vi "Fc_2update_graph.vi"(9 "Cluster in":T1, 10 "Local Mode":enum32{"Resume", "Hold"}(ring), 11 "WaveformGraph in":refnum<vi>) -> (2 "Cluster in 2":T1, 3 "Update Waveform Graph":bool)   [LabVIEW 2021]
doc: "This function updates the waveform graph."
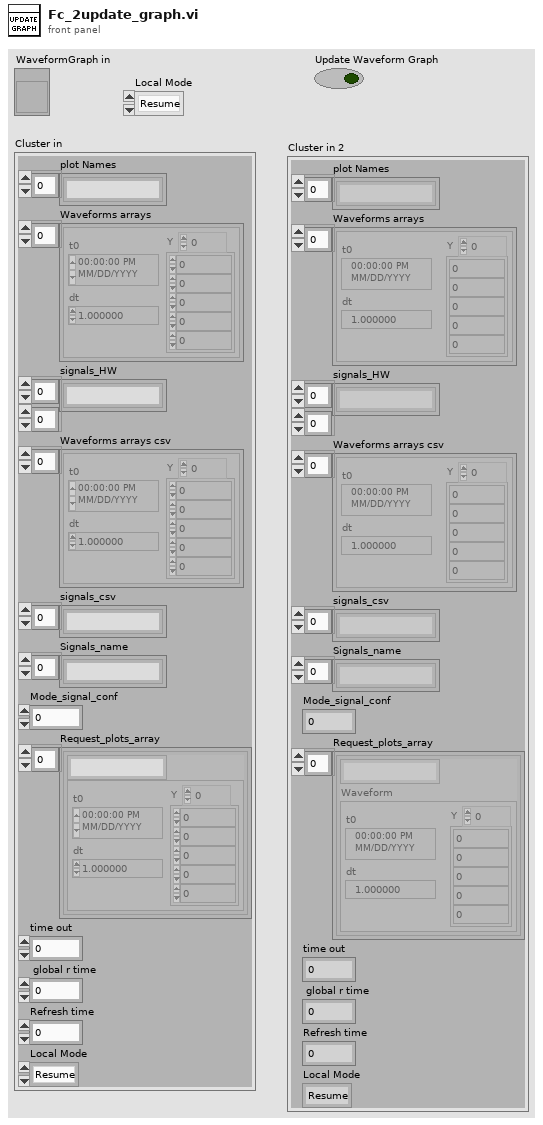
[diagram p1: front panel]
types:
  T1 = cluster{"plot Names":string[], "Waveforms arrays":waveform(dbl)[], "signals_HW":string[][], "Waveforms arrays csv":waveform(dbl)[], "signals_csv":string[], "Signals_name":string[], "Mode_signal_conf":u8, "Request_plots_array":cluster{string, "Waveform":waveform(dbl)}[], "time out":i32, " global r time":u32, "Refresh time":u32, "Local Mode":enum32{"Resume", "Hold"}}
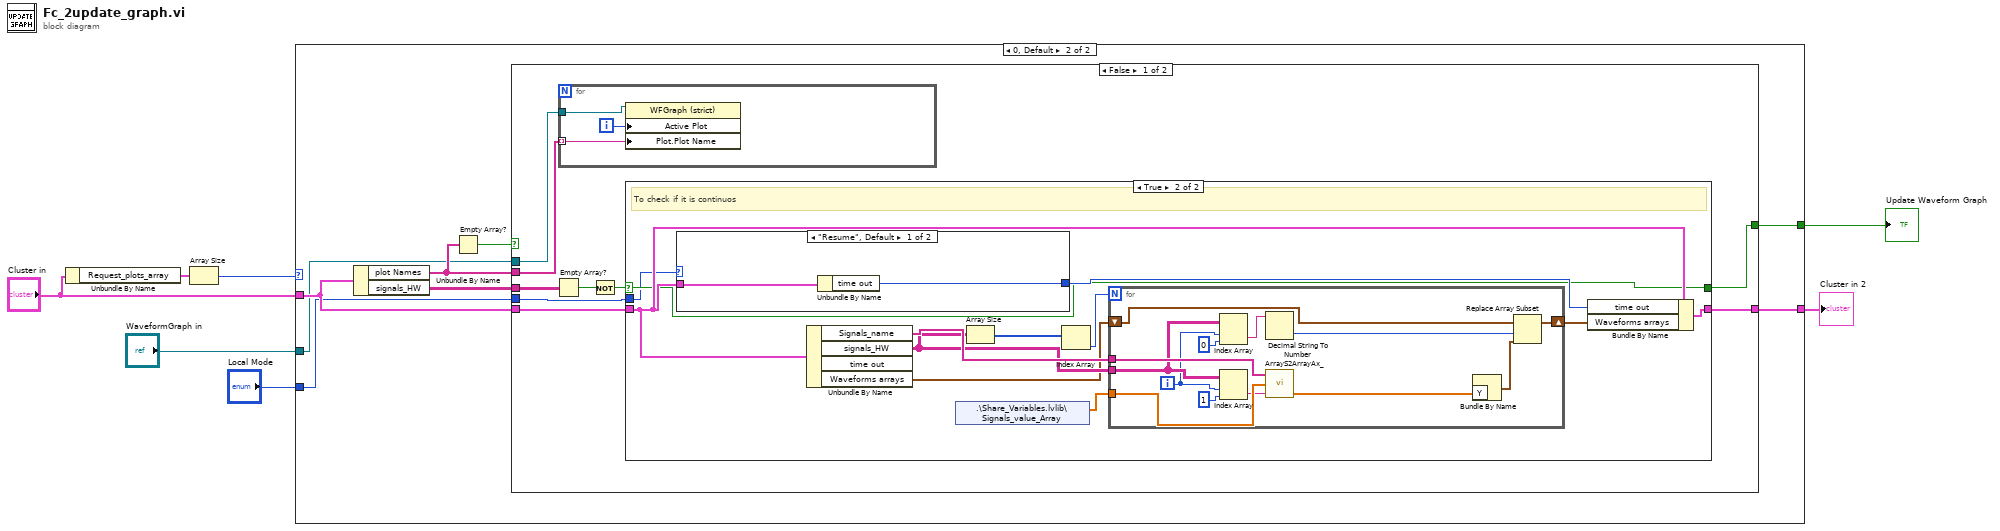
[diagram p0: block diagram]
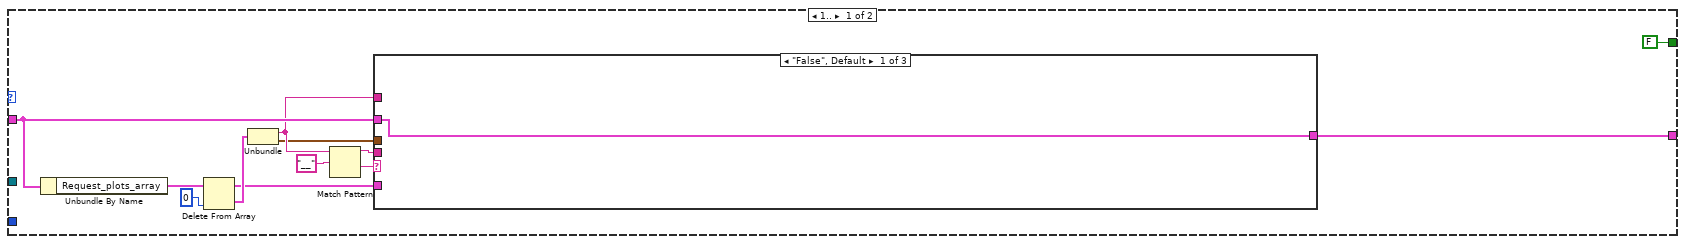
[diagram p2: hidden frame]
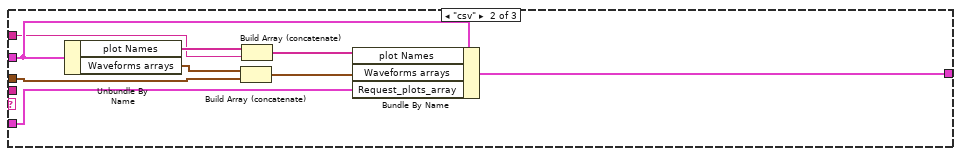
[diagram p3: hidden frame]
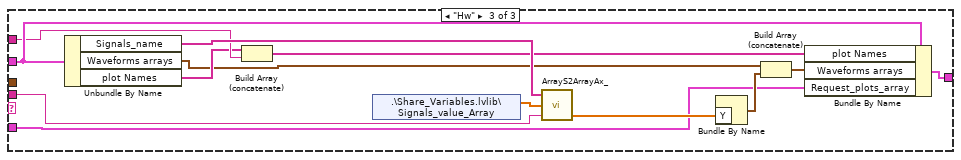
[diagram p4: hidden frame]
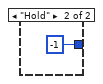
[diagram p6: hidden frame]
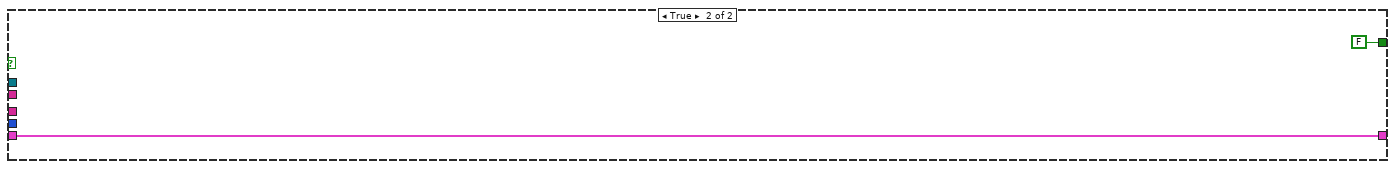
[diagram p7: hidden frame]
diagram:
  n1 = Unbundle By Name("Cluster in") -> ("Request_plots_array"=w4:cluster{string, "Waveform":waveform(dbl)}[])
  n2 = Array Size(array=w4) -> (size(s)=w5:i32)
  n3 = case shown="0, Default" w5 {
    tunnel: "Cluster in" -> [w15 w48]
    tunnel: [w16 w47] -> w6
    tunnel: [FALSE w45] -> w7
    tunnel: "WaveformGraph in" -> [_ w44]
    tunnel: "Local Mode" -> [_ w43]
    frame 1.. {
      n4 = Unbundle By Name(w15) -> ("Request_plots_array"=w10:cluster{string, "Waveform":waveform(dbl)}[])
      n5 = Delete From Array(array=w10, index=0) -> (deleted portion=w11:cluster{string, "Waveform":waveform(dbl)}, array with subset deleted=w9:cluster{string, "Waveform":waveform(dbl)}[])  [unwired: 1 in]
      n6 = Unbundle(w11) -> (w13:string, "Waveform"=w12:waveform(dbl))
      n7 = Match Pattern(string=w13, regular expression="__") -> (before substring=w17:string, after substring=w18:string)  [unwired: 1 in, 2 out]
      n8 = case shown="\"False\", Default" w18 {
        tunnel: w15 -> [w20 w29 w38]
        tunnel: w17 -> [_ _ w40]
        tunnel: w12 -> [_ w26 _]
        tunnel: w13 -> [_ w24 w37]
        tunnel: [w20 w22 w33] -> w16
        tunnel: w9 -> [_ w21 w31]
        frame "False", Default {
        }
        frame "csv" {
          n9 = Unbundle By Name(w29) -> ("plot Names"=w28:string[], "Waveforms arrays"=w27:waveform(dbl)[])
          n10 = Build Array (concatenate)(w27, w26) -> (w25:waveform(dbl)[])
          n11 = Build Array (concatenate)(w28, w24) -> (w23:string[])
          n12 = Bundle By Name(cluster=w29, "plot Names"=w23, "Waveforms arrays"=w25, "Request_plots_array"=w21) -> (w22:T1)
        }
        frame "Hw" {
          n13 = Unbundle By Name(w38) -> ("Signals_name"=w41:string[], "Waveforms arrays"=w30:waveform(dbl)[], "plot Names"=w32:string[])
          n14 = Build Array (concatenate)(w32, w37) -> (w36:string[])
          n15 = shared-variable ".\\Share_Variables.lvlib\\Signals_value_Array"() -> (w42:dbl[])  [unwired: 1 in, 1 out]
          n16 = call "ArrayS2ArrayAx_.vi"("Signal_input"=w40, "Signals_value_Array"=w42, "Signals_name"=w41) -> ("Subarray 1x_out"=w39:sgl[])  [unwired: 2 out]
          n17 = Bundle By Name("Y"=w39) -> (w35:waveform(sgl))  [unwired: 1 in]
          n18 = Build Array (concatenate)(w30, w35) -> (w34:waveform(dbl)[])
          n19 = Bundle By Name(cluster=w38, "plot Names"=w36, "Waveforms arrays"=w34, "Request_plots_array"=w31) -> (w33:T1)
        }
      }
    }
    frame 0, Default {
      n20 = Unbundle By Name(w48) -> ("plot Names"=w50:string[], "signals_HW"=w46:string[][])
      n21 = Empty Array?(array=w50) -> (empty?=w49:bool)
      n22 = case shown="False" w49 {
        tunnel: w50 -> [w59 _]
        tunnel: w46 -> [w57 _]
        tunnel: w48 -> [w58 w94]
        tunnel: [w54 w94] -> w47
        tunnel: [w53 FALSE] -> w45
        tunnel: w44 -> [w52 _]
        tunnel: w43 -> [w51 _]
        frame False {
          n23 = Empty Array?(array=w57) -> (empty?=w56:bool)
          n24 = for {
            tunnel: w59 -> [w91] mode=indexing
            tunnel: w52 -> [w90]
            i -> [w92]
            n25 = property on="Property Node" class="WFGraph (strict)"(reference=w90, "Active Plot"=w92, "Plot.Plot Name"=w91) -> ()  [unwired: 1 in, 2 out]
          }
          n26 = Not(x=w56) -> (.not. x?=w55:bool)
          n27 = case shown="True" w55 {
            selector: w55 -> [w60 w63]
            tunnel: w58 -> [w61 w64]
            tunnel: [w61 w67] -> w54
            tunnel: [w60 w63] -> w53
            tunnel: w51 -> [_ w62]
            frame False {
            }
            frame True {
              # "To check if it is continuos"
              n28 = case shown="\"Resume\", Default" w62 {
                tunnel: [w74 -1 ("time out")] -> w66
                tunnel: w64 -> [w75 _]
                frame "Resume", Default {
                  n29 = Unbundle By Name(w75) -> ("time out"=w74:i32)
                }
                frame "Hold" {
                }
              }
              n30 = Unbundle By Name(w64) -> ("Signals_name"=w72:string[], "signals_HW"=w71:string[][], "Waveforms arrays"=w68:waveform(dbl)[])  [unwired: 1 out]
              n31 = shared-variable ".\\Share_Variables.lvlib\\Signals_value_Array"() -> (w73:dbl[])  [unwired: 1 in, 1 out]
              n32 = Array Size(array=w71) -> (size(s)=w70:i32[])
              n33 = Index Array(array=w70) -> (element=w69:i32)  [unwired: 1 in]
              n34 = for {
                N: w69 -> [_]
                tunnel: w71 -> [w87]
                tunnel: w73 -> [w89]
                tunnel: w72 -> [w88]
                shift-right: [w77] -> w65
                shift-left: w68 -> [w82]
                i -> [w79]
                n35 = Index Array(array=w87, index (row)=w79, index (col)=0 ("disabled index (row)")) -> (element=w85:string)
                n36 = Index Array(array=w87, index (row)=w79, index (col)=1 ("index")) -> (element=w86:string)
                n37 = Decimal String To Number(string=w85) -> (number=w81:i32)  [unwired: 2 in, 1 out]
                n38 = call "ArrayS2ArrayAx_.vi"("Signal_input"=w86, "Signals_value_Array"=w89, "Signals_name"=w88) -> ("Subarray 1x_out"=w84:sgl[])  [unwired: 2 out]
                n39 = Bundle By Name("Y"=w84) -> (w83:waveform(sgl))  [unwired: 1 in]
                n40 = Replace Array Subset(array=w82, new element=w83, index=w81) -> (w77:waveform(dbl)[])
              }
              n41 = Bundle By Name(cluster=w64, "time out"=w66, "Waveforms arrays"=w65) -> (w67:T1)
            }
          }
        }
        frame True {
        }
      }
    }
  }
  "Update Waveform Graph" <- w7
  "Cluster in 2" <- w6
